vi "Get Multi.vi"(0 "Display State In":T20, 5 "Value In":T1={"Type"=enum."Tone", "Tone"={"Frequency (kHz)"=0.0, "Phase (cycles)"=0.0, "Random phase"=FALSE}, "Pulse Train"={"Pulse width (us)"=0.0, "Pulse rate (Hz)"=0.0, "Gap (ms)"=0.0, "Polarity"=enum."POS", "PT State"={"Template"=[], "Nperiod"=0, "Index"=0, "Pulse Rate (Hz)"=0.0, "Phase (cycles)"=0.0, "Noff"=0}, "Asynch"=FALSE}, "Noise"={"Properties"={"InvFilt"=FALSE, "Aweight"=FALSE, "Seed"=0, "Tokens"=0, "Brickwall"=FALSE}, "Data"={"TokenNum"=0}}, "File"={"Filename"=path "", "Signal"=[], "Channel"=0, "stream"=FALSE, "offset"=0, "nreps"=0, "loops"=0, "Tokens"=0, "Randomize"=FALSE, "order"=[]}, "FMSweep"={"Rate (oct/s)"=0.0, "Fmin (Hz)"=0.0, "Fmax (Hz)"=0.0, "Ramp (ms)"=0.0, "Linear"=FALSE}, "Chirp Train"={"Params"={"Fmin (kHz)"=4.0, "Fmax (kHz)"=64.0, "Compensate"=FALSE, "Duration (ms)"=2.0}, "Data"={"WF"=[]}}, "Complex Tone"={"Params"={"F0 (Hz)"=0.0, "Band"={"Flow (Hz)"=0.0, "Fhigh (Hz)"=0.0}, "Phase"=enum."Cosine", "Min F0 (Hz)"=0.0, "Max F0 (Hz)"=0.0, "ContinRandPhase"=FALSE, "Max peak factor"=inf, "Max mod depth"=2.0, "MinHarmNum"=0, "MaxHarmNum"=0, "Level Mode"=enum."per component", "% jitter"=0.0}, "Data"={"Ncomp"=0, "MinHarm"=0, "Phase"=[], "Amplitude"=[], "Npts/frame"=0, "Last F0"=0.0, "Fmin"=0.0, "Fmax"=0.0, "Lslope"=0.0, "randphase"=FALSE, "overall rms"=FALSE, "fmult"=[], "jittered"=FALSE}}, "FM"={"Carrier (kHz)"=0.0, "ModRate (Hz)"=0.0, "Depth (Hz)"=0.0, "Phase (cycles)"=0.0}, "Vowel"={"Freqs"="", "Set level"=enum."Total", "Freq"=[], "weights"=[]}, "Ramp"={"Duration (ms)"=0.0}}, 9 "Container State":T22, 11 "error in (no error)":errorcluster) -> (4 "Display State Out":T20, 6 "Value Out":T1={"Type"=enum."Tone", "Tone"={"Frequency (kHz)"=0.0, "Phase (cycles)"=0.0, "Random phase"=FALSE}, "Pulse Train"={"Pulse width (us)"=0.0, "Pulse rate (Hz)"=0.0, "Gap (ms)"=0.0, "Polarity"=enum."POS", "PT State"={"Template"=[], "Nperiod"=0, "Index"=0, "Pulse Rate (Hz)"=0.0, "Phase (cycles)"=0.0, "Noff"=0}, "Asynch"=FALSE}, "Noise"={"Properties"={"InvFilt"=FALSE, "Aweight"=FALSE, "Seed"=0, "Tokens"=0, "Brickwall"=FALSE}, "Data"={"TokenNum"=0}}, "File"={"Filename"=path "", "Signal"=[], "Channel"=0, "stream"=FALSE, "offset"=0, "nreps"=0, "loops"=0, "Tokens"=0, "Randomize"=FALSE, "order"=[]}, "FMSweep"={"Rate (oct/s)"=0.0, "Fmin (Hz)"=0.0, "Fmax (Hz)"=0.0, "Ramp (ms)"=0.0, "Linear"=FALSE}, "Chirp Train"={"Params"={"Fmin (kHz)"=4.0, "Fmax (kHz)"=64.0, "Compensate"=FALSE, "Duration (ms)"=2.0}, "Data"={"WF"=[]}}, "Complex Tone"={"Params"={"F0 (Hz)"=0.0, "Band"={"Flow (Hz)"=0.0, "Fhigh (Hz)"=0.0}, "Phase"=enum."Cosine", "Min F0 (Hz)"=0.0, "Max F0 (Hz)"=0.0, "ContinRandPhase"=FALSE, "Max peak factor"=inf, "Max mod depth"=2.0, "MinHarmNum"=0, "MaxHarmNum"=0, "Level Mode"=enum."per component", "% jitter"=0.0}, "Data"={"Ncomp"=0, "MinHarm"=0, "Phase"=[], "Amplitude"=[], "Npts/frame"=0, "Last F0"=0.0, "Fmin"=0.0, "Fmax"=0.0, "Lslope"=0.0, "randphase"=FALSE, "overall rms"=FALSE, "fmult"=[], "jittered"=FALSE}}, "FM"={"Carrier (kHz)"=0.0, "ModRate (Hz)"=0.0, "Depth (Hz)"=0.0, "Phase (cycles)"=0.0}, "Vowel"={"Freqs"="", "Set level"=enum."Total", "Freq"=[], "weights"=[]}, "Ramp"={"Duration (ms)"=0.0}}, 15 "error out":errorcluster)   [LabVIEW 2015, in "Waveform (G3).xctl"]
uses:
  Waveform (G3).xctl
  <vilib>/_xctls/Container State.ctl
  State.ctl
  Utility VIs/Controls/KRing/KRing.xctl
  Tone (G3)/Tone (G3).xctl
  Noise (G3)/Noise (G3).xctl
  Noise (G3)/Noise (G3) - Persistent.ctl
  Waveform Data.ctl
  Waveform VIs/Waveform Enum (V3).ctl
  Tone (G3)/Tone.Properties.ctl
  Waveform VIs/Pulse Train VIs/Pulse Train Params.ctl
  Waveform VIs/Pulse Train VIs/Pulse Polarity.ctl
  Waveform VIs/Pulse Train VIs/PT-Continuous State.ctl
  Waveform VIs/Noise VIs/Noise (G3).ctl
  Waveform VIs/Noise VIs/Noise (G3).Properties.ctl
  Waveform VIs/Noise VIs/Noise (G3).Data.ctl
  Waveform VIs/File VIs/StimFile-Params.ctl
  Waveform VIs/FM Sweep VIs/FM Sweep Params.ctl
  Waveform VIs/Chirp Train VIs/Chirp Train.ctl
  Waveform VIs/Chirp Train VIs/Chirp Train Params.ctl
  Waveform VIs/Complex Tone VIs/CT-Params.ctl
  Waveform VIs/Complex Tone VIs/CT-Phase Enum.ctl
  Waveform VIs/Complex Tone VIs/CT-Runtime Data.ctl
  FM Tone/Data.ctl
  Vowel/Vowel.Properties.ctl
  Waveform VIs/Ramp VIs/Ramp.Properties.ctl
  <vilib>/_xctls/XControlSupport.lvlib
  FM Tone/FM Tone.xctl
  Vowel/Vowel.xctl
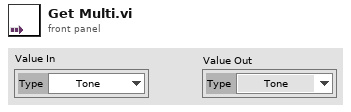
[diagram p1: front panel]
types:
  T1 = typedef "Waveform (G3).xctl/Waveform Data.ctl" = cluster{"Type":T2, "Tone":T3, "Pulse Train":T4, "Noise":T7, "File":T10, "FMSweep":T11, "Chirp Train":T12, "Complex Tone":cluster{"Params":T14, "Data":T16}, "FM":T17, "Vowel":T18, "Ramp":T19}
  T2 = typedef "Waveform Enum (V3).ctl" = enum16{"OFF", "Tone", "Noise", "Pulse Train", "File", "FM Sweep", "Chirp Train", "Complex Tone", "FM Tone", "Vowel", "Ramp"}
  T3 = typedef "Tone (G3).xctl/Tone.Properties.ctl" = cluster{"Frequency (kHz)":dbl, "Phase (cycles)":dbl, "Random phase":bool}
  T4 = typedef "Pulse Train Params.ctl" = cluster{"Pulse width (us)":dbl, "Pulse rate (Hz)":dbl, "Gap (ms)":dbl, "Polarity":T5, "PT State":T6, "Asynch":bool}
  T5 = typedef "Pulse Polarity.ctl" = enum16{"POS", "NEG", "POS-NEG", "NEG-POS"}
  T6 = typedef "PT-Continuous State.ctl" = cluster{"Template":dbl[], "Nperiod":i32, "Index":i32, "Pulse Rate (Hz)":dbl, "Phase (cycles)":dbl, "Noff":i32}
  T7 = typedef "Noise (G3).ctl" = cluster{"Properties":T8, "Data":T9}
  T8 = typedef "Noise (G3).Properties.ctl" = cluster{"InvFilt":bool, "Aweight":bool, "Seed":i32, "Tokens":i32, "Brickwall":bool}
  T9 = typedef "Noise (G3).Data.ctl" = cluster{"TokenNum":i32}
  T10 = typedef "StimFile-Params.ctl" = cluster{"Filename":path, "Signal":dbl[], "Channel":i32, "stream":bool, "offset":i32, "nreps":i32, "loops":i32, "Tokens":i32, "Randomize":bool, "order":i32[]}
  T11 = typedef "FM Sweep Params.ctl" = cluster{"Rate (oct/s)":dbl, "Fmin (Hz)":dbl, "Fmax (Hz)":dbl, "Ramp (ms)":dbl, "Linear":bool}
  T12 = typedef "Chirp Train.ctl" = cluster{"Params":T13, "Data":cluster{"WF":dbl[]}}
  T13 = typedef "Chirp Train Params.ctl" = cluster{"Fmin (kHz)":dbl, "Fmax (kHz)":dbl, "Compensate":bool, "Duration (ms)":dbl}
  T14 = typedef "CT-Params.ctl" = cluster{"F0 (Hz)":dbl, "Band":cluster{"Flow (Hz)":dbl, "Fhigh (Hz)":dbl}, "Phase":T15, "Min F0 (Hz)":dbl, "Max F0 (Hz)":dbl, "ContinRandPhase":bool, "Max peak factor":dbl, "Max mod depth":dbl, "MinHarmNum":i32, "MaxHarmNum":i32, "Level Mode":enum16{"per component", "overall rms"}, "% jitter":dbl}
  T15 = typedef "CT-Phase Enum.ctl" = enum16{"Cosine", "Random", "Alternating"}
  T16 = typedef "CT-Runtime Data.ctl" = cluster{"Ncomp":i32, "MinHarm":i32, "Phase":dbl[], "Amplitude":dbl[], "Npts/frame":i32, "Last F0":dbl, "Fmin":dbl, "Fmax":dbl, "Lslope":dbl, "randphase":bool, "overall rms":bool, "fmult":dbl[], "jittered":bool}
  T17 = typedef "FM Tone.xctl/Data.ctl" = cluster{"Carrier (kHz)":dbl, "ModRate (Hz)":dbl, "Depth (Hz)":dbl, "Phase (cycles)":dbl}
  T18 = typedef "Vowel.xctl/Vowel.Properties.ctl" = cluster{"Freqs":string, "Set level":enum16{"Total", "Per component"}, "Freq":dbl[], "weights":dbl[]}
  T19 = typedef "Ramp.Properties.ctl" = cluster{"Duration (ms)":dbl}
  T20 = typedef "Waveform (G3).xctl/State.ctl" = cluster{"Waveform names":string[], "Valid":bool[], "enable menu":bool, "Controls":cluster{"Type ":refnum<vi>, "Tone ":refnum<vi>, "Noise":refnum<vi>}, "persistent":cluster{"noise":T21, "Sort":bool}, "multi":bool}
  T21 = typedef "Noise (G3).xctl/Noise (G3) - Persistent.ctl" = cluster{"Show Aweight":bool}
  T22 = typedef "XControlSupport.lvlib/Container State.ctl" = cluster{"Indicator?":bool, "Run Mode?":bool, " Refnum":refnum<vi>}
  T23 = cluster{"Type ":refnum<vi>, "Tone ":refnum<vi>, "Noise":refnum<vi>}
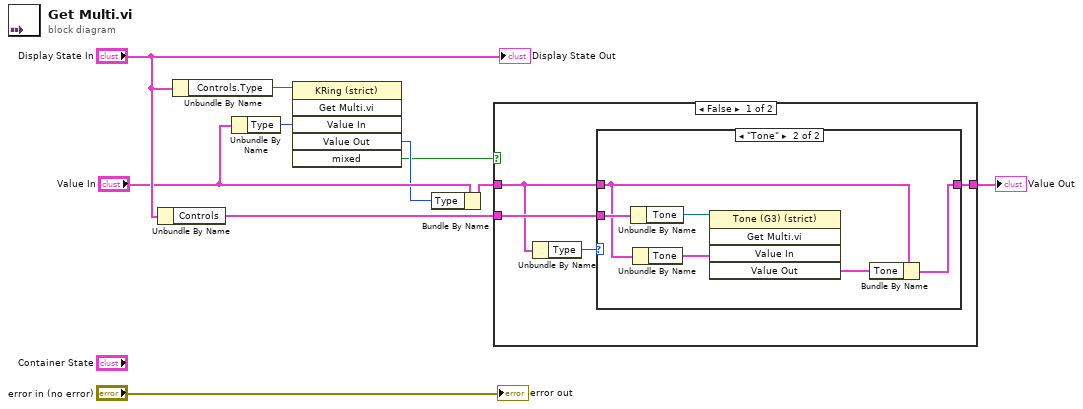
[diagram p0: block diagram]
diagram:
  n1 = Unbundle By Name("Display State In") -> ("Controls"=w8:T23)
  n2 = Unbundle By Name("Display State In") -> ("Controls.Type"=w6:refnum<vi>)
  n3 = Unbundle By Name("Value In") -> ("Type"=w5:T2)
  n4 = invoke class="KRing (strict)" method="Get Multi.vi"(reference=w6, "Value In"=w5) -> ("Value Out"=w2:i16, "mixed"=w1:bool)  [unwired: 4 in, 4 out]
  n5 = Bundle By Name(cluster="Value In", "Type"=w2) -> (w3:T1)
  n6 = case shown="False" w1 {
    tunnel: w3 -> [w11 w22]
    tunnel: [w12 w22] -> w9
    tunnel: w8 -> [w13 _]
    frame False {
      n7 = Unbundle By Name(w11) -> ("Type"=w14:T2)
      n8 = case shown="\"Tone\"" w14 {
        tunnel: w13 -> [_ w21]
        tunnel: w11 -> [w15 w18]
        tunnel: [w15 w17] -> w12
        frame "OFF", Default {
        }
        frame "Tone" {
          n9 = Unbundle By Name(w21) -> ("Tone"=w20:refnum<vi>)
          n10 = Unbundle By Name(w18) -> ("Tone"=w19:T3)
          n11 = invoke class="Tone (G3) (strict)" method="Get Multi.vi"(reference=w20, "Value In"=w19) -> ("Value Out"=w16:T3)  [unwired: 3 in, 4 out]
          n12 = Bundle By Name(cluster=w18, "Tone"=w16) -> (w17:T1)
        }
      }
    }
    frame True {
    }
  }
  "Value Out" <- w9
  "Display State Out" <- "Display State In"
  "error out" <- "error in (no error)"
